vi "AoRaster.vi"(0 "N":i32, 1 "Xoff":dbl format="%.3g", 2 "Frequency":dbl format="%.3g", 3 "Amplitude":dbl format="%.3g", 4 "On / Off":bool=TRUE, 5 "Yoff":dbl format="%.3g", 7 "AO Index":i32, 9 "error in (no error)":errorcluster) -> (6 "error out":errorcluster)   [LabVIEW 2009]
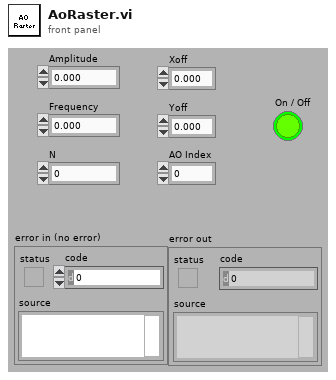
[diagram p1: front panel]
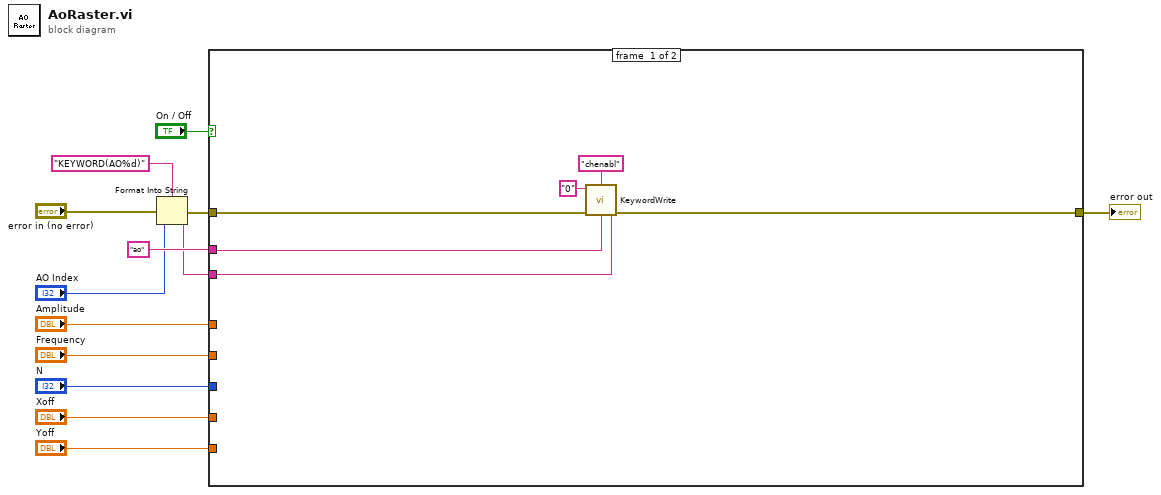
[diagram p0: block diagram]
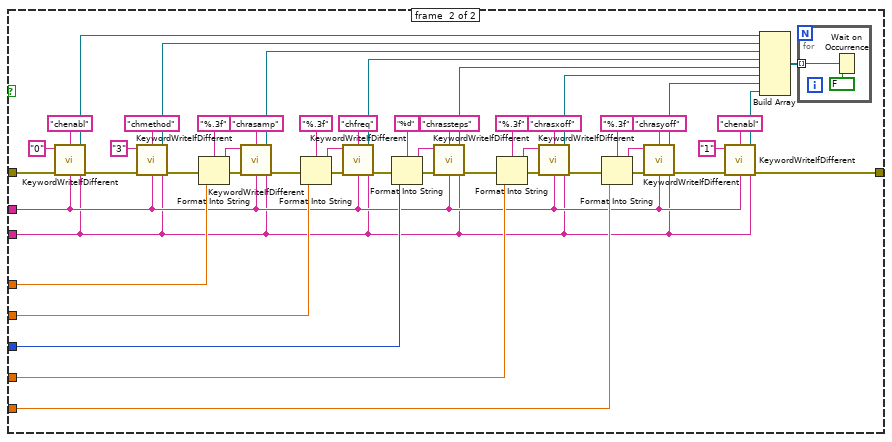
[diagram p2: hidden frame]
diagram:
  n1 = Format Into String(format string="KEYWORD(AO%d)", error in="error in (no error)", "AO Index") -> (resulting string=w8:string, error out=w3:errorcluster)  [unwired: 1 in]
  n2 = case shown="True" "On / Off" {
    tunnel: "Amplitude" -> [_ w69]
    tunnel: "Frequency" -> [_ w60]
    tunnel: w3 -> [w14 w46]
    tunnel: "N" -> [_ w53]
    tunnel: "ao" ("Service") -> [w15 w32]
    tunnel: w8 -> [w16 w31]
    tunnel: [w17 w50] -> w6
    tunnel: "Xoff" -> [_ w39]
    tunnel: "Yoff" -> [_ w33]
    frame #0 {
      n3 = call "KeywordWrite.vi"("Crate"=w16, "Keyword"="chenabl", "Value"="0", "Service"=w15, "error in (no error)"=w14) -> ("error out"=w17:errorcluster)  [unwired: 4 out]
    }
    frame #1 {
      n4 = call "KeywordWriteIfDifferent.vi"("Crate"=w31, "Keyword"="chenabl", "Value"="0", "Service"=w32, "error in (no error)"=w46) -> ("done?"=w28:refnum<k4>, "error out"=w45:errorcluster)  [unwired: 3 out]
      n5 = call "KeywordWriteIfDifferent.vi"("Crate"=w31, "Keyword"="chmethod", "Value"="3", "Service"=w32, "error in (no error)"=w45) -> ("done?"=w27:refnum<k4>, "error out"=w52:errorcluster)  [unwired: 3 out]
      n6 = Format Into String(format string="%.3f", error in=w52, w69) -> (resulting string=w67:string, error out=w66:errorcluster)  [unwired: 1 in]
      n7 = call "KeywordWriteIfDifferent.vi"("Crate"=w31, "Keyword"="chrasamp", "Value"=w67, "Service"=w32, "error in (no error)"=w66) -> ("done?"=w26:refnum<k4>, "error out"=w61:errorcluster)  [unwired: 3 out]
      n8 = Format Into String(format string="%.3f", error in=w61, w60) -> (resulting string=w64:string, error out=w65:errorcluster)  [unwired: 1 in]
      n9 = call "KeywordWriteIfDifferent.vi"("Crate"=w31, "Keyword"="chfreq", "Value"=w64, "Service"=w32, "error in (no error)"=w65) -> ("done?"=w25:refnum<k4>, "error out"=w54:errorcluster)  [unwired: 3 out]
      n10 = Format Into String(format string="%d", error in=w54, w53) -> (resulting string=w56:string, error out=w55:errorcluster)  [unwired: 1 in]
      n11 = call "KeywordWriteIfDifferent.vi"("Crate"=w31, "Keyword"="chrassteps", "Value"=w56, "Service"=w32, "error in (no error)"=w55) -> ("done?"=w24:refnum<k4>, "error out"=w40:errorcluster)  [unwired: 3 out]
      n12 = Format Into String(format string="%.3f", error in=w40, w39) -> (resulting string=w43:string, error out=w44:errorcluster)  [unwired: 1 in]
      n13 = call "KeywordWriteIfDifferent.vi"("Crate"=w31, "Keyword"="chrasxoff", "Value"=w43, "Service"=w32, "error in (no error)"=w44) -> ("done?"=w23:refnum<k4>, "error out"=w34:errorcluster)  [unwired: 3 out]
      n14 = Format Into String(format string="%.3f", error in=w34, w33) -> (resulting string=w36:string, error out=w35:errorcluster)  [unwired: 1 in]
      n15 = call "KeywordWriteIfDifferent.vi"("Crate"=w31, "Keyword"="chrasyoff", "Value"=w36, "Service"=w32, "error in (no error)"=w35) -> ("done?"=w22:refnum<k4>, "error out"=w30:errorcluster)  [unwired: 3 out]
      n16 = call "KeywordWriteIfDifferent.vi"("Crate"=w31, "Keyword"="chenabl", "Value"="1", "Service"=w32, "error in (no error)"=w30) -> ("done?"=w21:refnum<k4>, "error out"=w50:errorcluster)  [unwired: 3 out]
      n17 = Build Array(w28, w27, w26, w25, w24, w23, w22, w21) -> (w20:refnum<k4>[])
      n18 = for {
        tunnel: w20 -> [w71] mode=indexing
        n19 = Wait on Occurrence(1:FALSE ("ignore previous (T)"), 2:w71) -> ()  [unwired: 2 out]
      }
    }
  }
  "error out" <- w6
